vi "libtiff2_writeScanLine_U16m.vi"(7 "totalpages":i32, 8 "error in (no error)":errorcluster, 9 "page":u32, 10 "Data":u16[][](array[numeric]), 11 "Handle":i32) -> (0 "error out":errorcluster, 3 "Handle out":i32)   [LabVIEW 2012]
doc: "Write a (U16) page using LIBTIFFwriteScanLine to a file previously open for writing"
uses:
  C:/Program Files (x86)/GnuWin32/bin/libtiff3.dll
panel:
  out "status_compression":i32
  out "status width":i32
  out "status_length":i32
  out "status_spp":i32
  out "status_bps":i32
  out "status_orientation":i32
  out "status_planarconfig":i32
  out "status_photo":i32
  out "status_writscanline":i32
  out "status_subfile":i32
  out "status_writedir":i32
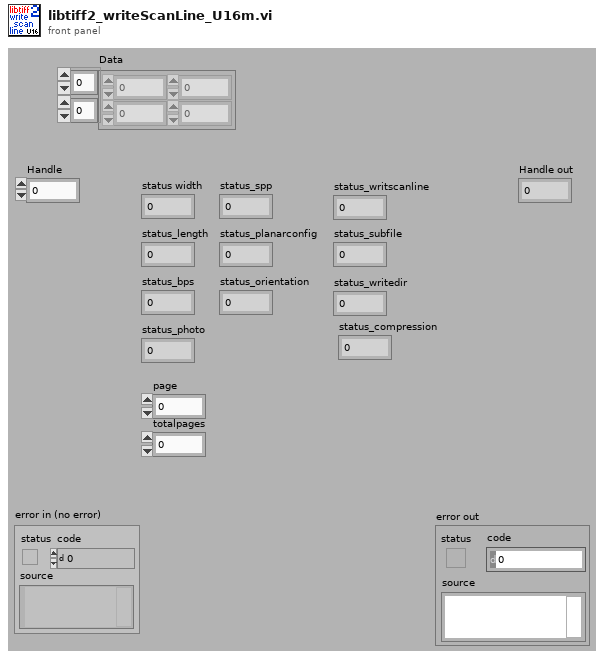
[diagram p1: front panel]
types:
  T1 = enum16{"Vertical flip", "Horizontal flip", "transpose", "rotate 90", "rotate 180", "rotate 270", "Diagonal flip"}
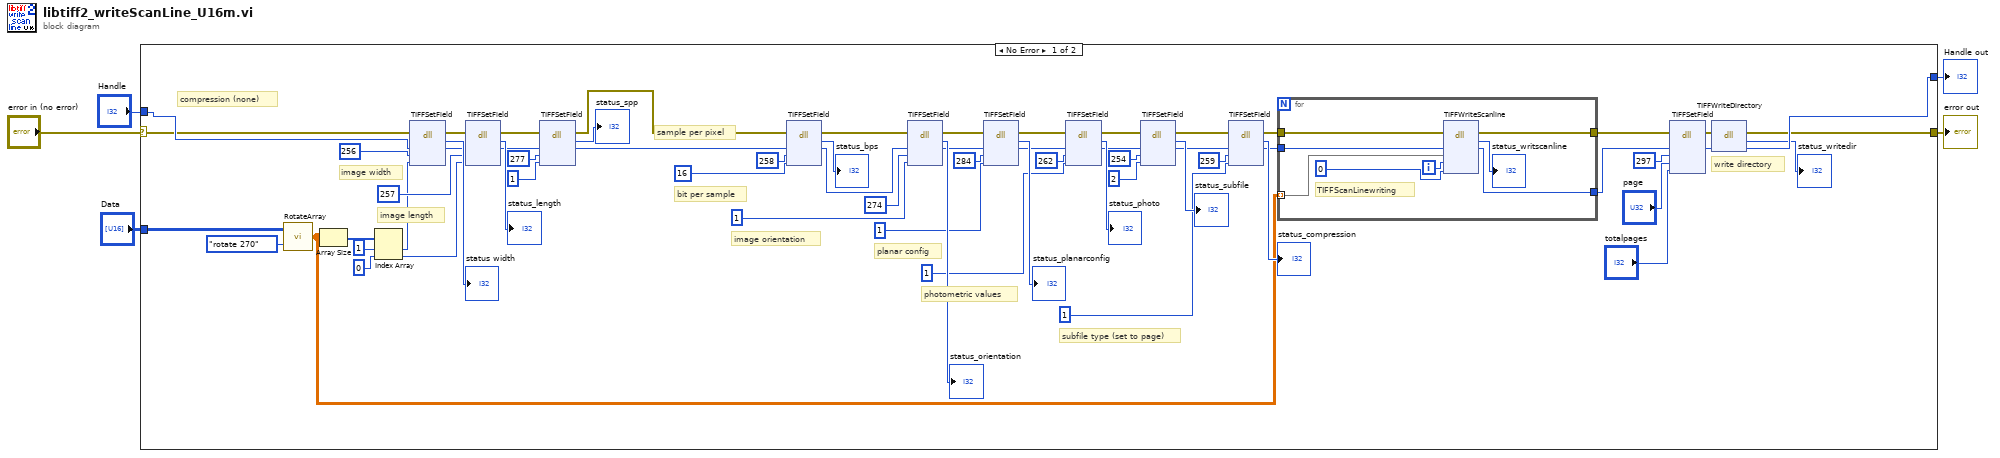
[diagram p0: block diagram]
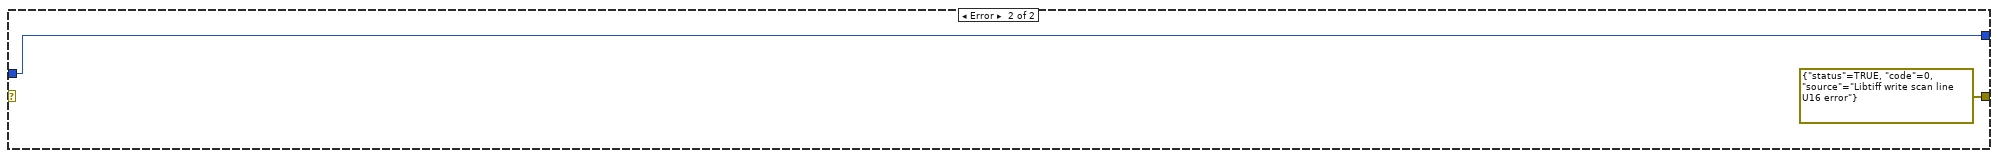
[diagram p2: hidden frame]
diagram:
  n1 = case shown="No Error" "error in (no error)" {
    selector: "error in (no error)" -> [w65 _]
    tunnel: "Handle" -> [w68 w78]
    tunnel: [w67 w78] -> w4
    tunnel: [w66 errorcluster {"status"=TRUE, "code"=0, "source"="Libtiff write scan line U16 error"} ("error out")] -> w3
    tunnel: "Data" -> [w64 _]
    frame No Error {
      # "compression (none)"
      # "write directory"
      # "subfile type (set to page)"
      # "photometric values"
      # "planar config"
      # "image orientation"
      # "bit per sample"
      # "sample per pixel"
      # "image length"
      # "image width"
      n2 = call "RotateArray.vi"("Method"=T1."rotate 270", "Input"=w64) -> ("Output"=w6:dbl[][])
      n3 = Array Size(array=w6) -> (size(s)=w32:i32[])
      n4 = Index Array(array=w32, index #1=1 ("index"), index #2=0 ("index")) -> (element #1=w17:i32, element #2=w18:i32)
      n5 = dll-call lib="C:/Program Files (x86)/GnuWin32/bin/libtiff3.dll" fn="TIFFSetField"(error in=w65, "Handle"=w68, "TIFF_tag"=256, "Value"=w17) -> (error out=w27:errorcluster, →"status width":i32, "Handle"=w61:i32)  [unwired: 4 in, 1 out]
      n6 = dll-call lib="C:/Program Files (x86)/GnuWin32/bin/libtiff3.dll" fn="TIFFSetField"(error in=w27, "Handle"=w61, "TIFF_tag"=257, "value"=w18) -> (error out=w26:errorcluster, →"status_length":i32, "Handle"=w58:i32)  [unwired: 4 in, 1 out]
      n7 = dll-call lib="C:/Program Files (x86)/GnuWin32/bin/libtiff3.dll" fn="TIFFSetField"(error in=w26, "Handle"=w58, "TIFF_tag"=277, "value"=u32 1) -> (error out=w25:errorcluster, →"status_spp":i32, "Handle"=w55:i32)  [unwired: 4 in, 1 out]
      n8 = dll-call lib="C:/Program Files (x86)/GnuWin32/bin/libtiff3.dll" fn="TIFFSetField"(error in=w25, "Handle"=w55, "TIFF_tag"=258, "value"=u32 16) -> (error out=w24:errorcluster, →"status_bps":i32, "Handle"=w52:i32)  [unwired: 4 in, 1 out]
      n9 = dll-call lib="C:/Program Files (x86)/GnuWin32/bin/libtiff3.dll" fn="TIFFSetField"(error in=w24, "Handle"=w52, "TIFF_tag"=274, "value"=u32 1) -> (error out=w23:errorcluster, →"status_orientation":i32, "Handle"=w48:i32)  [unwired: 4 in, 1 out]
      n10 = dll-call lib="C:/Program Files (x86)/GnuWin32/bin/libtiff3.dll" fn="TIFFSetField"(error in=w23, "Handle"=w48, "TIFF_tag"=284, "value"=u32 1) -> (error out=w22:errorcluster, →"status_planarconfig":i32, "Handle"=w44:i32)  [unwired: 4 in, 1 out]
      n11 = dll-call lib="C:/Program Files (x86)/GnuWin32/bin/libtiff3.dll" fn="TIFFSetField"(error in=w22, "Handle"=w44, "TIFF_tag"=262, "value"=u32 1) -> (error out=w21:errorcluster, →"status_photo":i32, "Handle"=w39:i32)  [unwired: 4 in, 1 out]
      n12 = dll-call lib="C:/Program Files (x86)/GnuWin32/bin/libtiff3.dll" fn="TIFFSetField"(error in=w21, "Handle"=w39, "TIFF_tag"=254, "value"=u32 2) -> (error out=w20:errorcluster, →"status_subfile":i32, "Handle"=w29:i32)  [unwired: 4 in, 1 out]
      n13 = dll-call lib="C:/Program Files (x86)/GnuWin32/bin/libtiff3.dll" fn="TIFFSetField"(error in=w20, "Handle"=w29, "TIFF_tag"=259, "value"=u32 1) -> (error out=w16:errorcluster, →"status_compression":i32, "Handle"=w15:i32)  [unwired: 4 in, 1 out]
      n14 = for {
        tunnel: [w75] -> w10
        tunnel: [w74] -> w11
        tunnel: w15 -> [w72]
        tunnel: w16 -> [w73]
        tunnel: w6 -> [w69] mode=indexing
        i -> [w71]
        # "TIFFScanLinewriting"
        n15 = dll-call lib="C:/Program Files (x86)/GnuWin32/bin/libtiff3.dll" fn="TIFFWriteScanline"(error in=w73, "Handle"=w72, "buffer"=w69, "row"=w71, "sample"=0) -> (error out=w74:errorcluster, "return type"=→"status_writscanline":i32, "Handle"=w75:i32)  [unwired: 5 in, 1 out]
      }
      n16 = dll-call lib="C:/Program Files (x86)/GnuWin32/bin/libtiff3.dll" fn="TIFFSetField"(error in=w11, "Handle"=w10, "TIFF_tag"=297, "page"="page", "totalpages"="totalpages") -> (error out=w9:errorcluster, "Handle"=w8:i32)  [unwired: 5 in, 2 out]
      n17 = dll-call lib="C:/Program Files (x86)/GnuWin32/bin/libtiff3.dll" fn="TIFFWriteDirectory"(error in=w9, "Handle"=w8) -> (error out=w66:errorcluster, →"status_writedir":i32, "Handle"=w67:i32)  [unwired: 2 in, 1 out]
    }
    frame Error {
    }
  }
  "Handle out" <- w4
  "error out" <- w3
